vi "OAT Auto Range.vi"(6 "num of steps wanted":i32=200, 8 "posible increament":dbl[](array[numeric]) format="%.2f", 9 "lower limit":dbl format="%.2f", 10 "upper limit":dbl format="%.2f", 11 "range in":T1 {"Increment" format="%.2f"; "Maximum" format="%.2f"; "Minimum" format="%.2f"}) -> (2 "total step":i32, 3 "range out":T1 {"Increment" format="%.2f"; "Maximum" format="%.2f"; "Minimum" format="%.2f"})   [LabVIEW 2017]
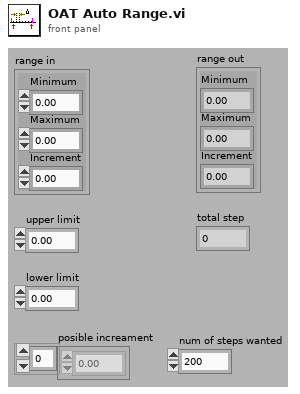
[diagram p1: front panel]
types:
  T1 = cluster{"Minimum":dbl, "Maximum":dbl, "Increment":dbl}
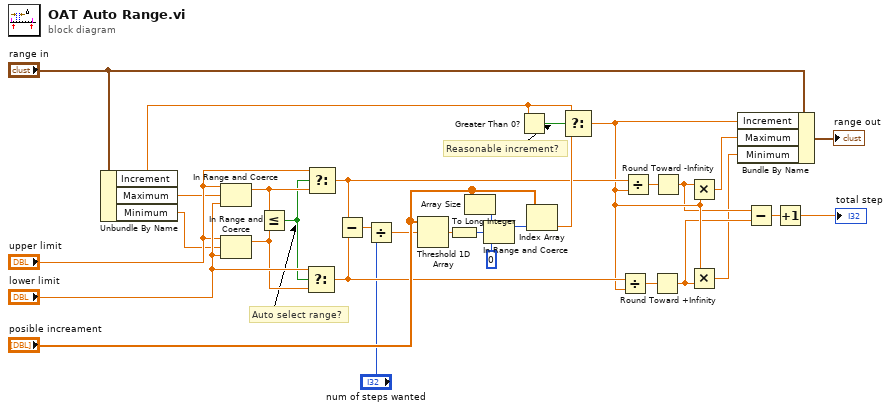
[diagram p0: block diagram]
diagram:
  # "Auto select range?"
  # "Reasonable increment?"
  n1 = Unbundle By Name("range in") -> ("Increment"=w22:dbl, "Maximum"=w13:dbl, "Minimum"=w14:dbl)
  n2 = In Range and Coerce(upper limit="upper limit", x=w13, lower limit="lower limit") -> (coerced(x)=w18:dbl)  [unwired: 1 out]
  n3 = In Range and Coerce(upper limit="upper limit", x=w14, lower limit="lower limit") -> (coerced(x)=w19:dbl)  [unwired: 1 out]
  n4 = Less Or Equal?(x=w18, y=w19) -> (x <= y?=w12:bool)
  n5 = Select(t="lower limit", s=w12, f=w19) -> (s? t:f=w20:dbl)
  n6 = Select(t="upper limit", s=w12, f=w18) -> (s? t:f=w21:dbl)
  n7 = Subtract(x=w21, y=w20) -> (x-y=w10:dbl)
  n8 = Divide(x=w10, y="num of steps wanted") -> (x/y=w23:dbl)
  n9 = Threshold 1D Array(2:w23, 3:"posible increament") -> (0:w27:dbl)  [unwired: 1 in]
  n10 = To Long Integer(number=w27) -> (32bit integer=w28:i32)
  n11 = Array Size(array="posible increament") -> (size(s)=w24:i32)
  n12 = In Range and Coerce(upper limit=w24, x=w28, lower limit=0) -> (coerced(x)=w26:i32)  [unwired: 1 out]
  n13 = Greater Than 0?(x=w22) -> (x > 0?=w5:bool)
  n14 = Index Array(array="posible increament", index=w26) -> (element=w29:dbl)
  n15 = Select(t=w22, s=w5, f=w29) -> (s? t:f=w16:dbl)
  n16 = Divide(x=w20, y=w16) -> (x/y=w2:dbl)
  n17 = Divide(x=w21, y=w16) -> (x/y=w3:dbl)
  n18 = Round Toward +Infinity(x=w2) -> (ceil(x): smallest int >= x=w15:dbl)
  n19 = Round Toward -Infinity(1:w3) -> (0:w9:dbl)
  n20 = Multiply(x=w9, y=w16) -> (x*y=w17:dbl)
  n21 = Multiply(x=w16, y=w15) -> (x*y=w8:dbl)
  n22 = Bundle By Name(cluster="range in", "Increment"=w16, "Maximum"=w17, "Minimum"=w8) -> (→"range out":T1)
  n23 = Subtract(x=w9, y=w15) -> (x-y=w6:dbl)
  n24 = Increment(x=w6) -> (x+1=→"total step":dbl)
